vi "Comsetting.vi"(3 "error in":errorcluster, 4 "HardwareSetting":T1, 5 "Enum":enum16{"read", "write"}(ring)=enum."write") -> (0 "error our":errorcluster, 1 "HardwareSetting":T1, 2 "appended path 2":path)   [LabVIEW 2017]
doc: "VI for saving Hardware setting for PLC IP and Camera IP address. an PORT"
uses:
  <vilib>/Utility/config.llb/NI_LVConfig.lvlib
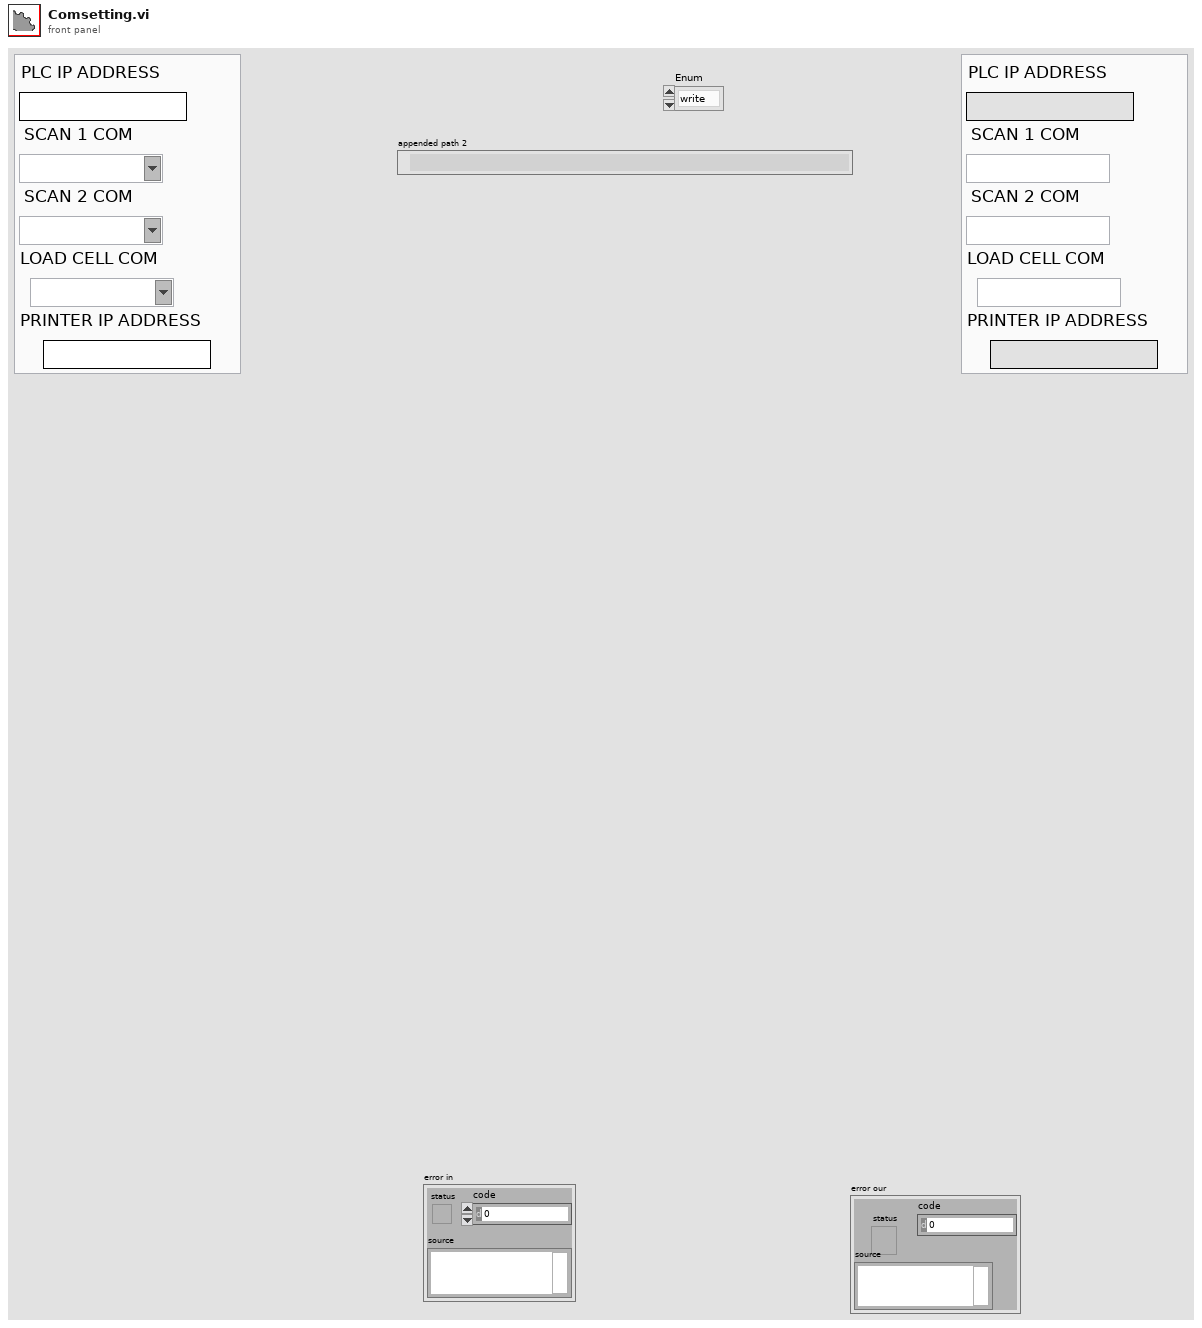
[diagram p1: front panel]
types:
  T1 = cluster{"PLC IP ADDRESS":string, "SCAN 1 COM":refnum<visa-resource-name>, "SCAN 2 COM":refnum<visa-resource-name>, "LOAD CELL COM":refnum<visa-resource-name>, "PRINTER IP ADDRESS":string}
  T2 = enum32{"invalid app kind", "Development System", "Run Time System", "Student Edition", "Embedded LabVIEW", "Evaluation", "Custom"}
  T3 = typedef "NI_LVConfig.lvlib/Config Data RefNum.ctl" = refnum<k1>
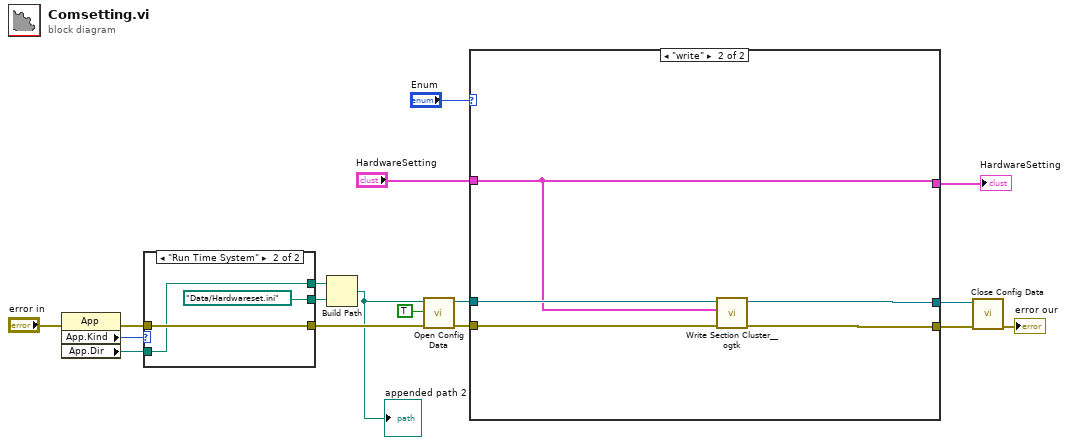
[diagram p0: block diagram]
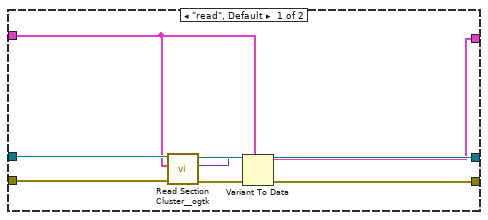
[diagram p2: hidden frame]
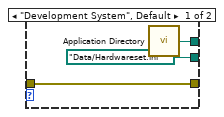
[diagram p3: hidden frame]
diagram:
  n1 = property class="App"(error in="error in") -> (error out=w10:errorcluster, "App.Kind"=w4:T2, "App.Dir"=w9:path)  [unwired: 1 in, 1 out]
  n2 = case shown="\"Run Time System\"" w4 {
    tunnel: [w20 w23] -> w11
    tunnel: w10 -> [w20 w23]
    tunnel: w9 -> [_ w21]
    tunnel: [path "Data/Hardwareset.ini" path "Data/Hardwareset.ini"] -> w8
    tunnel: [w18 w21] -> w7
    frame "Development System", Default {
      n3 = call <vilib>:"Application Directory.vi"() -> ("Application Directory"=w18:path)
    }
    frame "Run Time System" {
    }
  }
  n4 = Build Path(base path=w7, name or relative path=w8) -> (appended path=w6:path)
  "appended path 2" <- w6
  n5 = call <vilib>:"Open Config Data.vi"("error in (no error)"=w11, "create file if necessary (T)"=TRUE, "configuration file path"=w6) -> ("error out"=w16:errorcluster, "refnum"=w15:T3)  [unwired: 6 in, 1 out]
  n6 = case shown="\"write\"" "Enum" {
    tunnel: [w26 w34] -> w13
    tunnel: w16 -> [w31 w36]
    tunnel: w15 -> [w30 w35]
    tunnel: [w29 w33] -> w12
    tunnel: "HardwareSetting" -> [w24 w32]
    tunnel: [w25 w32] -> w1
    frame "read", Default {
      n7 = call <userlib>:"Read Section Cluster__ogtk.vi"("error in (no error)"=w31, "Section Formatted Cluster Type"=w24, "refnum"=w30) -> ("error out"=w27:errorcluster, "Section Formatted Cluster"=w28:variant, "dup refnum"=w29:T3)  [unwired: 4 in, 2 out]
      n8 = Variant To Data(error in=w27, type=w24, Variant=w28) -> (data=w25:T1, error out=w26:errorcluster)
    }
    frame "write" {
      n9 = call <userlib>:"Write Section Cluster__ogtk.vi"("error in (no error)"=w36, "Section Formatted Cluster"=w32, "refnum"=w35) -> ("error out"=w34:errorcluster, "dup refnum"=w33:T3)  [unwired: 7 in]
    }
  }
  "HardwareSetting" <- w1
  n10 = call <vilib>:"Close Config Data.vi"("error in (no error)"=w13, "refnum"=w12) -> ("error out"=→"error our":errorcluster)  [unwired: 8 in, 1 out]
